vi "ERD_Read_List_Builder.vi"(1 "ERD Read List ALL":T1=[{"Boolean"=TRUE, "ERD Number"=49, "ERD Name"="Build Number", "Data Type"=enum."uint32_t"}, {"Boolean"=TRUE, "ERD Number"=127, "ERD Name"="Build Hash", "Data Type"=enum."string"}] {"ERD Number" format="%.0x"}, 5 "Error In":errorcluster) -> (14 "Read ERD List":T2[](array[typedef]) {"ERD Number" format="%.0x"}, 16 "ERD Name":string[](array[string]), 19 "Error Out":errorcluster)   [LabVIEW 2023]
doc: "This VI takes an array of ERD Cluster Data. Cluster conatins a boolean to Read the ERD or not, ERD number, name, and data type. It the compiles an array of ERD data to use in ERD Read VI."
uses:
  LabVIEW GEA2 Toolkit/GEA3/type defs/ERD Read Data In.ctl
  type defs/ERD Read List All.ctl
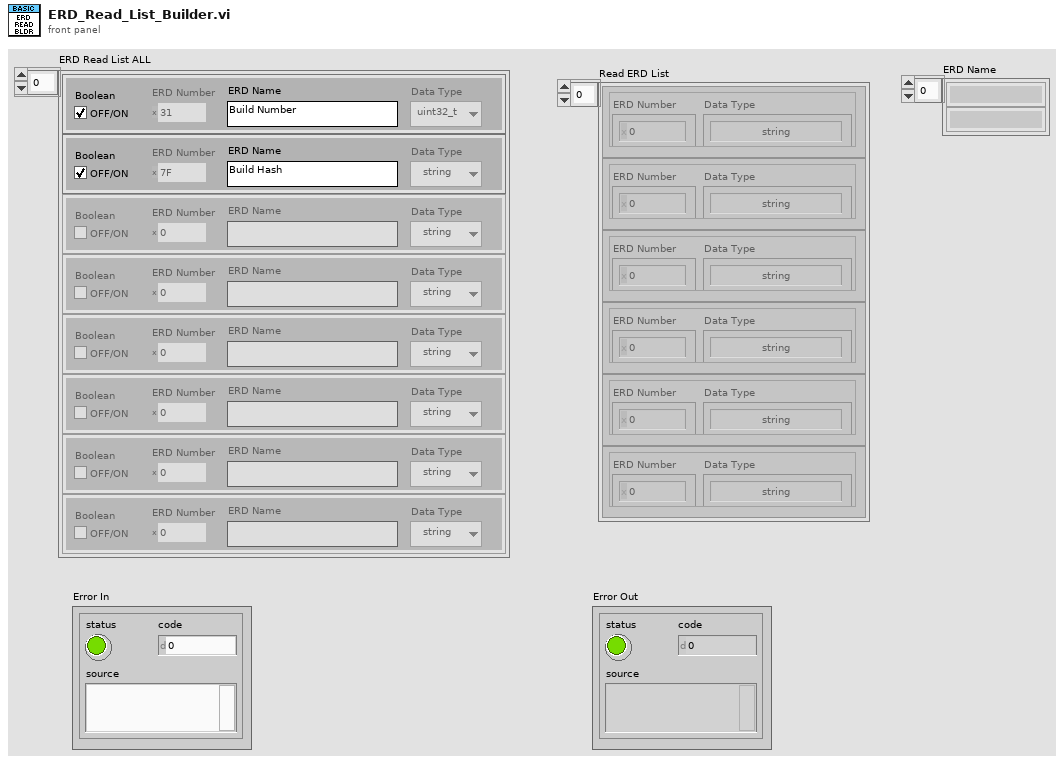
[diagram p1: front panel]
types:
  T1 = typedef "ERD Read List All.ctl" = cluster{"Boolean":bool, "ERD Number":u16, "ERD Name":string, "Data Type":enum16{"string", "boolean", "uint8_t", "uint16_t", "uint32_t", "uint64_t", "int8_t", "int16_t", "int32_t", "int64_t"}}[]
  T2 = typedef "ERD Read Data In.ctl" = cluster{"ERD Number":u16, "Data Type":enum16{"string", "boolean", "uint8_t", "uint16_t", "uint32_t", "uint64_t", "int8_t", "int16_t", "int32_t", "int64_t"}}
  T3 = enum16{"string", "boolean", "uint8_t", "uint16_t", "uint32_t", "uint64_t", "int8_t", "int16_t", "int32_t", "int64_t"}
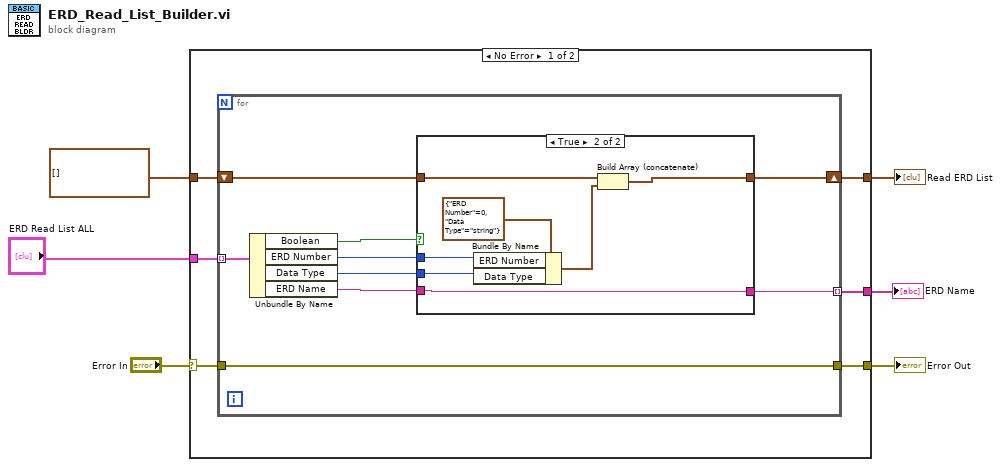
[diagram p0: block diagram]
diagram:
  n1 = case shown="No Error" "Error In" {
    selector: "Error In" -> [w9 w30]
    tunnel: "ERD Read List ALL" -> [w12 _]
    tunnel: [w11 _] -> w6
    tunnel: T2[] [] -> [w10 _]
    tunnel: [w8 w30] -> w3
    tunnel: [w7 _] -> w2
    frame No Error {
      n2 = for {
        tunnel: w12 -> [w21] mode=indexing
        shift-right: [w17] -> w11
        shift-left: w10 -> [w18]
        tunnel: w9 -> [w15]
        tunnel: [w15] -> w8
        tunnel: [w13] -> w7 mode=indexing
        n3 = Unbundle By Name(w21) -> ("Boolean"=w20:bool, "ERD Number"=w19:u16, "Data Type"=w16:T3, "ERD Name"=w14:string)
        n4 = case shown="True" w20 {
          tunnel: w19 -> [_ w24]
          tunnel: w18 -> [w22 w29]
          tunnel: [w22 w27] -> w17
          tunnel: w16 -> [_ w25]
          tunnel: w14 -> [_ w23]
          tunnel: [_ w23] -> w13
          frame False {
          }
          frame True {
            n5 = Bundle By Name(cluster=T2 {"ERD Number"=0, "Data Type"=enum."string"} ("ERD Read Data In"), "ERD Number"=w24, "Data Type"=w25) -> (w28:T2)
            n6 = Build Array (concatenate)(w29, w28) -> (w27:T2[])
          }
        }
      }
    }
    frame Error {
    }
  }
  "Read ERD List" <- w6
  "Error Out" <- w3
  "ERD Name" <- w2
